vi "GetOCUCommands.vi"(8 "error in (no error)":errorcluster, 9 "MissionArray":refnum<class "GenericMission.lvclass">[](array[class]), 10 "MissionToDelete":refnum<queue>, 11 "MissionFromOCU":refnum<queue>) -> (0 "error out":errorcluster, 3 "UpdatedMissionArray":refnum<class "GenericMission.lvclass">[](array[class]))   [LabVIEW 2013]
doc: "Add a mission or delets a misison from the CurrentMissions array when an item to add or delete is put into the respecitve queues"
uses:
  Logic/Classes/Missions/GenericMission/GenericMission.lvclass
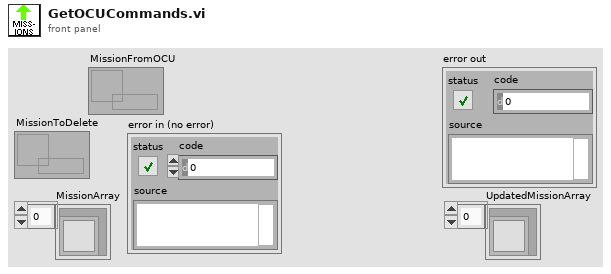
[diagram p1: front panel]
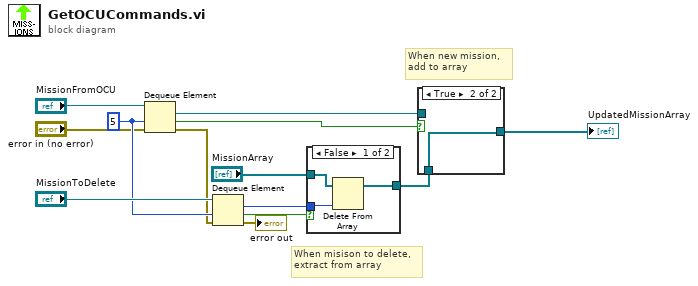
[diagram p0: block diagram]
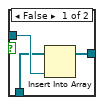
[diagram p3: hidden frame]
diagram:
  w12 = 5 ("timeout in ms (-1)")
  # "When new mission,\nadd to array"
  # "When misison to delete,\nextract from array"
  n1 = Dequeue Element(queue="MissionFromOCU", timeout in ms (-1)=w12, error in (no error)="error in (no error)") -> (element=w8:refnum<class "GenericMission.lvclass">, timed out?=w10:bool, error out=w4:errorcluster)  [unwired: 1 out]
  n2 = Dequeue Element(queue="MissionToDelete", timeout in ms (-1)=w12, error in (no error)=w4) -> (element=w9:i32, timed out?=w3:bool, error out=→"error out":errorcluster)  [unwired: 1 out]
  n3 = case shown="False" w3 {
    tunnel: "MissionArray" -> [w16 w17]
    tunnel: w9 -> [w15 _]
    tunnel: [w14 w17] -> w6
    frame False {
      n4 = Delete From Array(array=w16, index=w15) -> (array with subset deleted=w14:refnum<class "GenericMission.lvclass">[])  [unwired: 1 in, 1 out]
    }
    frame True {
    }
  }
  n5 = case shown="True" w10 {
    tunnel: w8 -> [w20 _]
    tunnel: w6 -> [w19 w21]
    tunnel: [w18 w21] -> w1
    frame False {
      n6 = Insert Into Array(array=w19, new element=w20) -> (w18:refnum<class "GenericMission.lvclass">[])  [unwired: 1 in]
    }
    frame True {
    }
  }
  "UpdatedMissionArray" <- w1
